vi "Serialize - JSON.vi"(8 "error in (no error)":errorcluster, 11 "2D Single Data in":refnum<class "2D Single Data.lvclass">) -> (0 "error out":errorcluster, 2 "Serialized JSON":string, 3 "2D Single Data out":refnum<class "2D Single Data.lvclass">)   [LabVIEW 2016, in "Base Data Class.lvlib" / "2D Single Data.lvclass"]
uses:
  2D Single Data.lvclass
  Data.lvclass
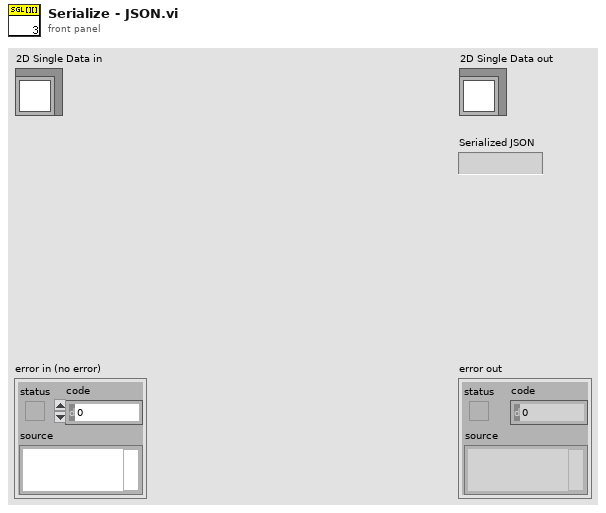
[diagram p1: front panel]
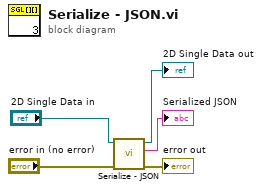
[diagram p0: block diagram]
diagram:
  n1 = call-parent "Serialize - JSON.vi"("error in"="error in (no error)", "Data in"="2D Single Data in") -> ("error out"=→"error out":errorcluster, "Serialized JSON"=→"Serialized JSON":string, "Data out"=→"2D Single Data out":refnum<class "2D Single Data.lvclass">)  [unwired: 7 in]
